vi "Read AI Data.vi"(8 "error in (no error)":errorcluster, 11 "DAQ Data in":refnum<class "DAQ Data.lvclass">) -> (0 "error out":errorcluster, 2 "AI Data":dbl[](array[numeric]), 3 "DAQ Data out":refnum<class "DAQ Data.lvclass">)   [LabVIEW 2022 SP3, in "DAQ Data.lvclass"]
uses:
  DAQ Data.lvclass
  DAQ Data.lvclass/DAQ Data.ctl
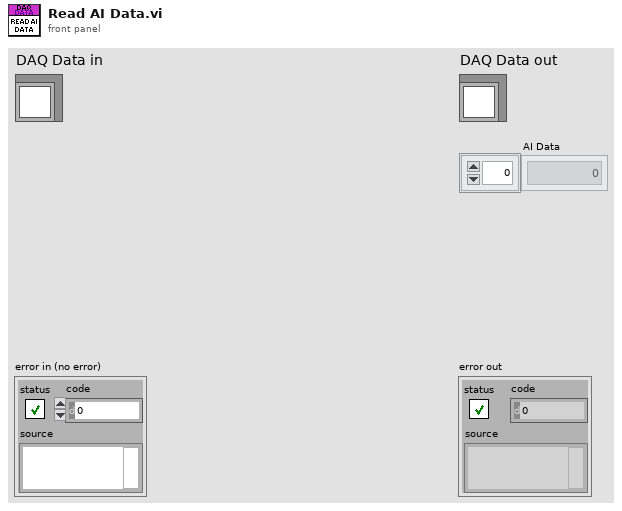
[diagram p1: front panel]
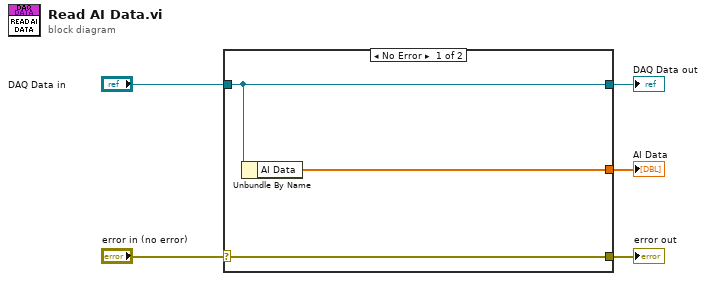
[diagram p0: block diagram]
diagram:
  n1 = case shown="No Error" "error in (no error)" {
    selector: "error in (no error)" -> [w8 w9]
    tunnel: [w8 w9] -> w4
    tunnel: [w7 w10] -> w2
    tunnel: "DAQ Data in" -> [w7 w10]
    tunnel: [w6 _] -> w1
    frame No Error {
      n2 = Unbundle By Name(w7) -> ("AI Data"=w6:dbl[])
    }
    frame Error {
    }
  }
  "error out" <- w4
  "DAQ Data out" <- w2
  "AI Data" <- w1
